vi "data check intensity_dataset.vi"() -> ()   [LabVIEW 2016]
uses:
  <vilib>/Utility/file.llb/Read Delimited Spreadsheet (DBL).vi
  <vilib>/Utility/file.llb/Write Delimited Spreadsheet (DBL).vi
panel:
  out "부분배열":dbl[](array[numeric])
  out "강도 그래프 2":dbl[][](graph)
  in  "file path":path caption="파일 경로(비었을 경우 대화 상자 창)"
  out "크기 2":i32
  out "output":dbl[](array[numeric])
  out "x*y":i32
  out "크기":i32[](array[numeric])
  in  "file path (dialog if empty)":path caption="파일 경로(비었을 경우 대화 상자 창)"
  out "강도 그래프":dbl[][](graph)
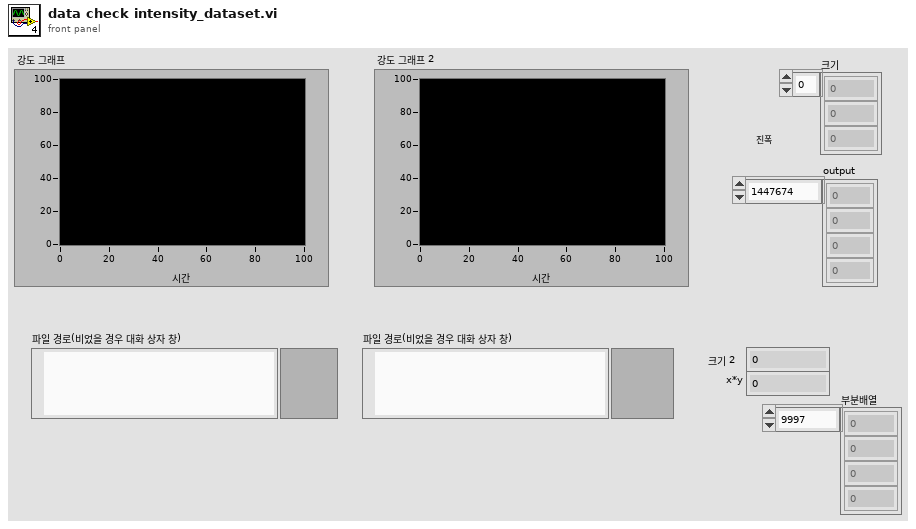
[diagram p1: front panel]
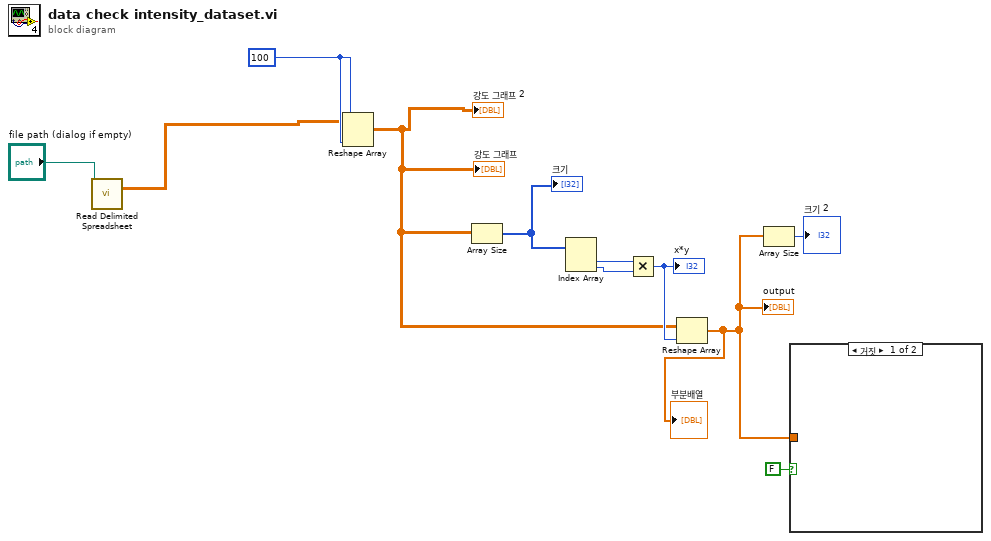
[diagram p0: block diagram]
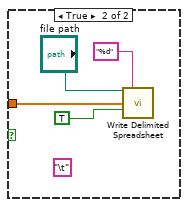
[diagram p2: hidden frame]
diagram:
  w4 = 100 ("차원 크기")
  n1 = call-poly <vilib>:"Read Delimited Spreadsheet.vi"("file path (dialog if empty)"="file path (dialog if empty)") -> ("all rows"=w2:dbl[][])  [unwired: 9 in, 5 out]
  n2 = Reshape Array(w2, w4, w4) -> (w3:dbl[][])
  "강도 그래프" <- w3
  "강도 그래프 2" <- w3
  n3 = Array Size(array=w3) -> (size(s)=w8:i32[])
  "크기" <- w8
  n4 = Index Array(array=w8) -> (element #1=w10:i32, element #2=w9:i32)  [unwired: 2 in]
  n5 = Multiply(x=w10, y=w9) -> (x*y=w7:i32)
  "x*y" <- w7
  n6 = Reshape Array(w3, w7) -> (w1:dbl[])
  "output" <- w1
  "부분배열" <- w1
  n7 = Array Size(array=w1) -> (size(s)=→"크기 2":i32)
  n8 = case shown="거짓" FALSE {
    tunnel: w1 -> [_ w15]
    frame False {
    }
    frame True {
      (unwired) "\t" ("delimiter (\\t)")
      n9 = call-poly <vilib>:"Write Delimited Spreadsheet.vi"("file path (dialog if empty)"="file path", "format (%.3f)"="%d", "1D data"=w15, "append to file? (new file:F)"=TRUE) -> ()  [unwired: 10 in, 2 out]
    }
  }
